vi "fpga_LP1 Process.vi"(0 "input data":fxp<+/-,32,3>, 1 "reset":bool, 5 "Ch":fxp<+,5,5>=6.0, 9 "input valid":bool, 12 "ready for output":bool) -> (4 "re":fxp<+/-,32,5> format="%.29g", 6 "im":fxp<+/-,32,5> format="%.29g", 10 "output valid":bool, 14 "ready for input":bool)   [LabVIEW 2011, in "NI_EP_PMU_FPGA.lvlib"]
uses:
  <vilib>/addons/Electrical Power/PMU/NI_EP_PMU_FPGA.lvlib
  <vilib>/rvi/DataTransferAndStorage/Container/Common/niFpgaContainerState.ctl
  <vilib>/rvi/DataTransferAndStorage/Container/Common/niFpgaDataTypeControl.ctl
  <vilib>/rvi/DataTransferAndStorage/Container/Common/niFpgaContainerImplementationControl.ctl
  <vilib>/rvi/DataTransferAndStorage/Container/Common/niFpgaContainerArbitrationOptionsControl.ctl
  <vilib>/rvi/DataTransferAndStorage/Container/Common/niFpgaTransferTypeControl.ctl
  <vilib>/rvi/DataTransferAndStorage/Container/Common/niFpgaContainerInitializationParameters.ctl
  <vilib>/rvi/Memory/Memory_Types/niFpgaMemoryInterfaceConfiguration.ctl
  <vilib>/rvi/FIFO/Fifo_Types/niFpgaFifoControlLogicControl.ctl
  <vilib>/rvi/DataTransferAndStorage/Container/Common/niFpgaContainerMetaDataKey.ctl
  <vilib>/rvi/DataTransferAndStorage/Container/Common/niFpgaContainerGetUniqueNameForEmu.vi
  <vilib>/rvi/DataTransferAndStorage/Container/Common/niFpgaContainerSetEmuInfo.vi
  <vilib>/rvi/eio/common/nirviEmuReportErrorAndStop.vi
  <vilib>/rvi/FIFO/Fifo_Resource/nirvififoEmulationSetSize.vi
  <vilib>/rvi/Memory/Memory_Emulation/niFpgaMemoryEmulationValidateCache.vi
  <vilib>/rvi/Memory/Memory_Emulation/nirvimemoryEmulationManagerCache_InsertValue.vi
  <vilib>/Utility/error.llb/Clear Errors.vi
  <vilib>/rvi/Memory/Memory_Emulation/nirvimemoryEmulationManagerCache_GetValue.vi
  <vilib>/rvi/LocalResourceManager/LocalResourceManager.xnode
  <vilib>/rvi/DataTransferAndStorage/Container/XNode/niFpgaContainer.xnode
  <vilib>/rvi/FIFO/Fifo_Resource/nirvififoEmulationRead.vi
  <vilib>/rvi/FXPMathLib/basic elements/FxpDiscreteDelay/XNode/nifxpmath_DiscreteDelay.xnode
  <vilib>/rvi/FXPMathLib/FxpMul/XNode/nifxpmath_Multiplier.xnode
  <vilib>/rvi/Memory/Memory_Emulation/nirvimemoryEmulation.vi
  <vilib>/rvi/FIFO/Fifo_Resource/nirvififoEmulationWrite.vi
  <vilib>/addons/Electrical Power/PQ/Resampling/NI_EP_Resample_FPGA.lvlib
  <vilib>/rvi/FXPMathLib/sim/FxpSim.dll
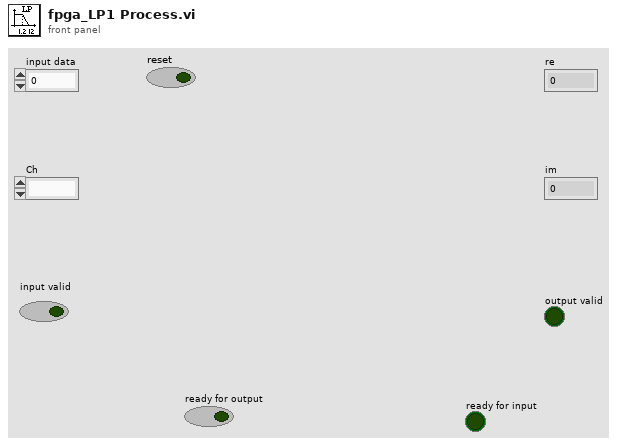
[diagram p1: front panel]
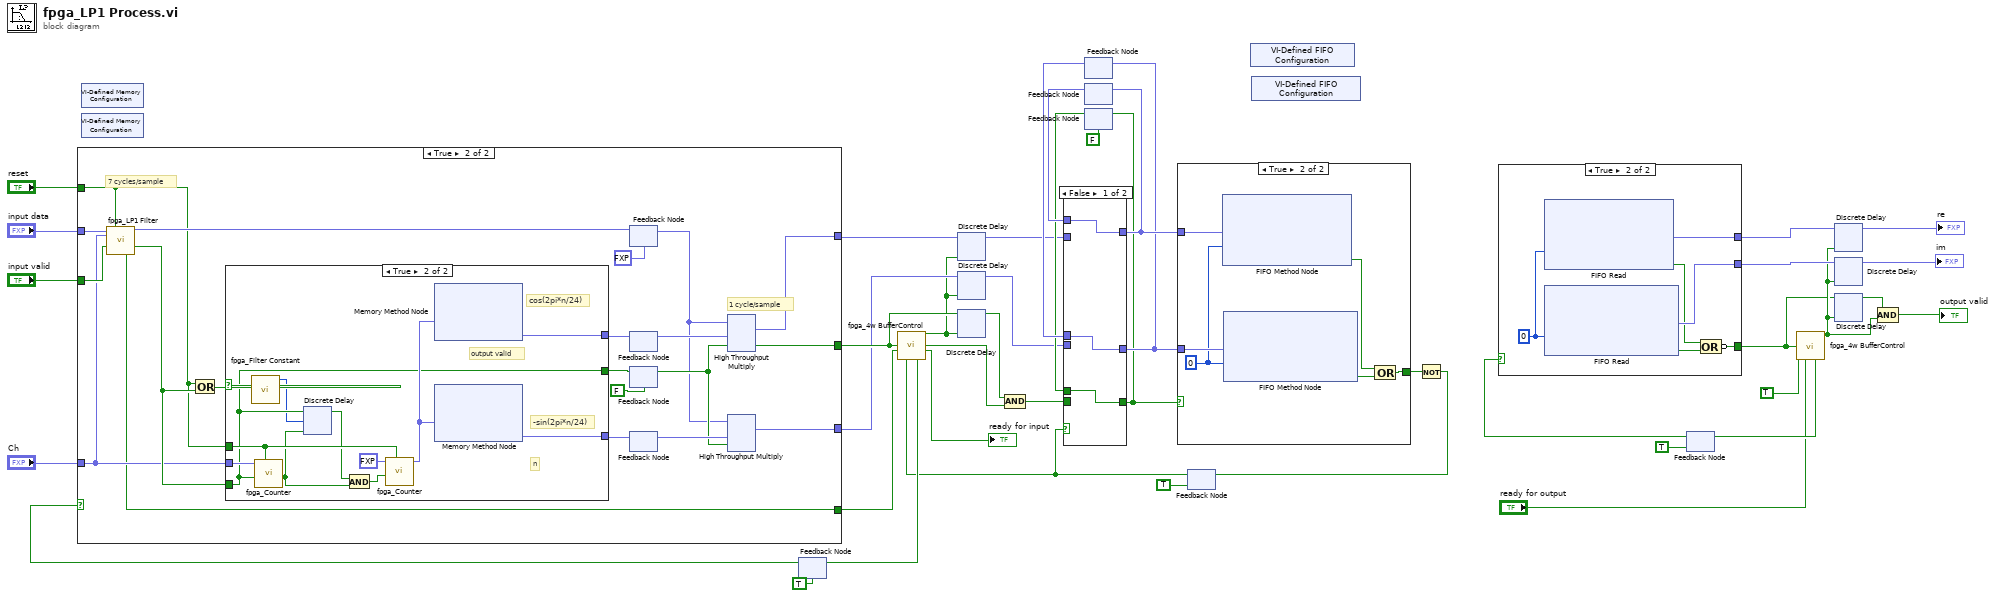
[diagram p0: block diagram]
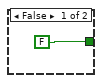
[diagram p6: hidden frame]
diagram:
  n1 = xnode "VI-Defined Memory Configuration"() -> ()  [unwired: 1 out]
  n2 = xnode "VI-Defined Memory Configuration"() -> ()  [unwired: 1 out]
  n3 = feedback #1(TRUE ("logic enable")) -> (w27:bool)
  n4 = case shown="True" w27 {
    tunnel: "input data" -> [_ w55]
    tunnel: "input valid" -> [_ w53]
    tunnel: "reset" -> [_ w50]
    tunnel: [_ w47] -> w7
    tunnel: [_ w43] -> w39
    tunnel: [_ w46] -> w6
    tunnel: [_ w45] -> w3
    tunnel: "Ch" -> [_ w44]
    frame False {
    }
    frame True {
      # "1 cycle/sample"
      # "7 cycles/sample"
      n5 = call <vilib>:"fpga_LP1 Filter.vi"("input data"=w55, "reset"=w50, "#Ch"=w44, "input valid"=w53) -> ("output data"=w54:fxp<+/-,32,4>, "output valid"=w51:bool, "ready for input"=w43:bool)  [unwired: 9 in]
      n6 = Or(x=w50, y=w51) -> (x .or. y?=w52:bool)
      n7 = case shown="True" w52 {
        tunnel: [_ w73] -> w56
        tunnel: [_ w74] -> w61
        tunnel: [FALSE w66] -> w59
        tunnel: w44 -> [_ w72]
        tunnel: w51 -> [_ w66]
        tunnel: w50 -> [_ w70]
        frame False {
        }
        frame True {
          # "-sin(2pi*n/24)"
          # "cos(2pi*n/24)"
          # "n"
          # "output valid"
          n8 = call <vilib>:"fpga_Filter Constant.vi"() -> ("LP1 delay"=w64:u8)  [unwired: 8 in, 3 out]
          n9 = call <vilib>:"fpga_Counter.vi"("reset"=w70, "Input Valid?"=w66, "upper limit"=w72) -> ("Multichannel Valid?"=w67:bool)  [unwired: 7 in, 1 out]
          n10 = xnode "Discrete Delay"("D"=w66, "n-1[0..15]"=w64, "enable"=w67) -> ("Q"=w65:bool)
          n11 = And(x=w65, y=w67) -> (x .and. y?=w71:bool)
          n12 = call <vilib>:"fpga_Counter.vi"("reset"=w70, "Input Valid?"=w71, "upper limit"=fxp<+,5,5> 24.0 ("#ch")) -> ("count"=w69:fxp<+,5,5>)  [unwired: 7 in, 1 out]
          n13 = xnode ("Memory Method Node")("Address"=w69) -> ("Data"=w73:fxp<+/-,32,2>)  [unwired: 1 in, 1 out]
          n14 = xnode ("Memory Method Node")("Address"=w69) -> ("Data"=w74:fxp<+/-,32,2>)  [unwired: 1 in, 1 out]
        }
      }
      n15 = feedback #2(fxp<+/-,32,4> 0.0 ("output data")) -> (w48:fxp<+/-,32,4>)
      n16 = feedback-in #2(w54) -> ()
      n17 = feedback #3() -> (w49:fxp<+/-,32,2>)  [unwired: 1 in]
      n18 = feedback-in #3(w56) -> ()
      n19 = feedback #4(FALSE) -> (w58:bool)
      n20 = feedback-in #4(w59) -> ()
      n21 = feedback #5() -> (w60:fxp<+/-,32,2>)  [unwired: 1 in]
      n22 = feedback-in #5(w61) -> ()
      n23 = xnode "High Throughput Multiply"("x"=w48, "y"=w49, "input valid"=w58) -> ("x*y"=w46:fxp<+/-,32,5>, "output valid"=w47:bool)  [unwired: 1 in, 1 out]
      n24 = xnode "High Throughput Multiply"("x"=w48, "y"=w60, "input valid"=w58) -> ("x*y"=w45:fxp<+/-,32,5>)  [unwired: 1 in, 2 out]
    }
  }
  n25 = feedback #6() -> (w37:fxp<+/-,32,5>)  [unwired: 1 in]
  n26 = feedback #7() -> (w38:fxp<+/-,32,5>)  [unwired: 1 in]
  n27 = feedback #8(FALSE) -> (w33:bool)
  n28 = feedback #9(TRUE) -> (w24:bool)
  n29 = call <vilib>:"fpga_4w BufferControl.vi"("DR"=w7, "RFI"=w39, "RFO"=w24) -> ("buff enable"=w2:bool, "output valid"=w30:bool, "ready for input"=→"ready for input":bool, "logic enable"=w28:bool)  [unwired: 9 in]
  n30 = feedback-in #1(w28) -> ()
  n31 = xnode "Discrete Delay"("D"=w6, "enable"=w2) -> ("Q"=w5:fxp<+/-,32,5>)
  n32 = xnode "Discrete Delay"("D"=w3, "enable"=w2) -> ("Q"=w1:fxp<+/-,32,5>)
  n33 = xnode "Discrete Delay"("D"=w7, "enable"=w2) -> ("Q"=w4:bool)
  n34 = Compound Arithmetic op=AND(w4, w30) -> (w31:bool)
  n35 = case shown="False" w24 {
    tunnel: w5 -> [_ w80]
    tunnel: w31 -> [_ w78]
    tunnel: w1 -> [_ w79]
    tunnel: [w77 w80] -> w36
    tunnel: w38 -> [w77 _]
    tunnel: [w76 w79] -> w29
    tunnel: w37 -> [w76 _]
    tunnel: [w75 w78] -> w12
    tunnel: w33 -> [w75 _]
    frame False {
    }
    frame True {
    }
  }
  n36 = feedback-in #6(w29) -> ()
  n37 = feedback-in #7(w36) -> ()
  n38 = feedback-in #8(w12) -> ()
  n39 = case shown="True" w12 {
    tunnel: w36 -> [_ w86]
    tunnel: w29 -> [_ w85]
    tunnel: [_ w81] -> w35
    frame False {
    }
    frame True {
      w84 = 0 ("Timeout")
      n40 = xnode ("FIFO Method Node")("Element"=w86, "Timeout"=w84) -> ("Timed Out?"=w82:bool)  [unwired: 1 in, 1 out]
      n41 = xnode ("FIFO Method Node")("Element"=w85, "Timeout"=w84) -> ("Timed Out?"=w83:bool)  [unwired: 1 in, 1 out]
      n42 = Compound Arithmetic op=OR(w82, w83) -> (w81:bool)
    }
  }
  n43 = xnode "VI-Defined FIFO Configuration"() -> ()  [unwired: 1 out]
  n44 = xnode "VI-Defined FIFO Configuration"() -> ()  [unwired: 1 out]
  n45 = Not(x=w35) -> (.not. x?=w8:bool)
  n46 = feedback-in #9(w8) -> ()
  n47 = feedback #10(TRUE ("logic enable")) -> (w21:bool)
  n48 = case shown="True" w21 {
    tunnel: [_ w92] -> w11
    tunnel: [_ w91] -> w18
    tunnel: [_ w89] -> w10
    frame False {
    }
    frame True {
      w90 = 0 ("Timeout")
      n49 = xnode ("FIFO Read")("Timeout"=w90) -> ("Element"=w89:fxp<+/-,32,5>, "Timed Out?"=w88:bool)  [unwired: 1 in, 1 out]
      n50 = xnode ("FIFO Read")("Timeout"=w90) -> ("Element"=w91:fxp<+/-,32,5>, "Timed Out?"=w87:bool)  [unwired: 1 in, 1 out]
      n51 = Compound Arithmetic op=OR(w88, w87) -> (invert w92:bool)
    }
  }
  n52 = call <vilib>:"fpga_4w BufferControl.vi"("DR"=w11, "RFI"=TRUE, "RFO"="ready for output") -> ("buff enable"=w13:bool, "logic enable"=w22:bool)  [unwired: 9 in, 2 out]
  n53 = feedback-in #10(w22) -> ()
  n54 = xnode "Discrete Delay"("D"=w10, "enable"=w13) -> ("Q"=→"re":fxp<+/-,32,5>)
  n55 = xnode "Discrete Delay"("D"=w18, "enable"=w13) -> ("Q"=→"im":fxp<+/-,32,5>)
  n56 = xnode "Discrete Delay"("D"=w11, "enable"=w13) -> ("Q"=w20:bool)
  n57 = Compound Arithmetic op=AND(w20, w13) -> (→"output valid":bool)
